vi "String to Hex.vi"(8 "error in":errorcluster, 11 "Insert_String":string) -> (0 "error out":errorcluster, 3 "Hex_String":string)   [LabVIEW 2020]
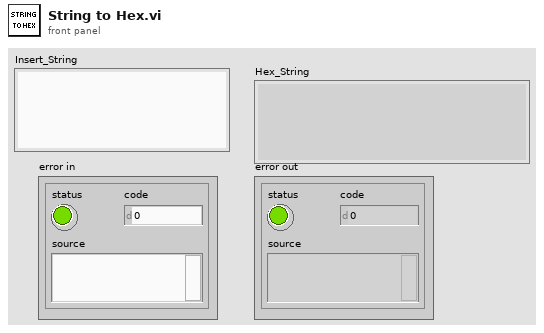
[diagram p1: front panel]
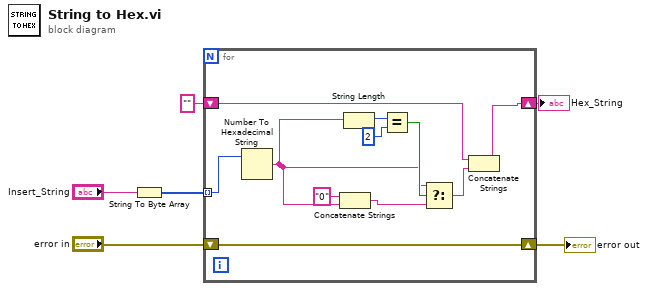
[diagram p0: block diagram]
diagram:
  n1 = String To Byte Array(string="Insert_String") -> (unsigned byte array=w5:u8[])
  n2 = for {
    tunnel: w5 -> [w9] mode=indexing
    shift-right: [w7] -> w4
    shift-left: "" -> [w8]
    shift-right: [w17] -> w2
    shift-left: "error in" -> [w17]
    n3 = Number To Hexadecimal String(2:w9) -> (0:w12:string)  [unwired: 1 in]
    n4 = Concatenate Strings("0" ("string"), w12) -> (w11:string)
    n5 = String Length(string=w12) -> (length=w16:i32)
    n6 = Equal?(x=w16, y=2) -> (x = y?=w14:bool)
    n7 = Select(t=w12, s=w14, f=w11) -> (s? t:f=w10:string)
    n8 = Concatenate Strings(w8, w10) -> (w7:string)
  }
  "Hex_String" <- w4
  "error out" <- w2
